vi "Fetch Waveform (Digital Waveform).vi"(4 "Ending Point (10000000)":i32=10000000, 6 "Starting Point (0)":i32, 8 "error in (no error)":errorcluster, 9 "Maximum Time (10000 ms)":u32=10000, 10 "Digital Channel (14: Digital Channel D0)":u16(ring)=14 items=["Digital Channel D0"=14, "Digital Channel D1"=15, "Digital Channel D2"=16, "Digital Channel D3"=17, "Digital Channel D4"=18, "Digital Channel D5"=19, "Digital Channel D6"=20, "Digital Channel D7"=21, "Digital Channel D8"=22, "Digital Channel D9"=23, "Digital Channel D10"=24, "Digital Channel D11"=25, "Digital Channel D12"=26, "Digital Channel D13"=27, "Digital Channel D14"=28, "Digital Channel D15"=29], 11 "VISA resource name":refnum<visa-resource-name>) -> (0 "error out":errorcluster, 2 "Digital Waveform":digitalwaveform(graph), 3 "VISA resource name out":refnum<visa-resource-name>)   [LabVIEW 2017, in "Tektronix DPO MSO 2000 4000 Series.lvlib"]
doc: "Fetches the digital waveform from the chosen digital channel. Please note that it might be necessary to increase the <B>Maximum Time</B> to approximately 170 seconds when fetching waveforms with 10 million data points.\n\n<B>Note:</B> This VI does not check the instrument status. Typically, you call this VI only in a sequence of calls to other low-level instrument driver VIs. The sequence performs one operation. You use the low-level VIs to optimize one or more aspects of interaction with the instrument. If you want to check the instrument status, call the <B>Error Query VI</B> at the conclusion of the sequence.\n\nLabVIEW versions higher than 7.1 might display the data differently."
uses:
  Tektronix DPO MSO 2000 4000 Series.lvlib
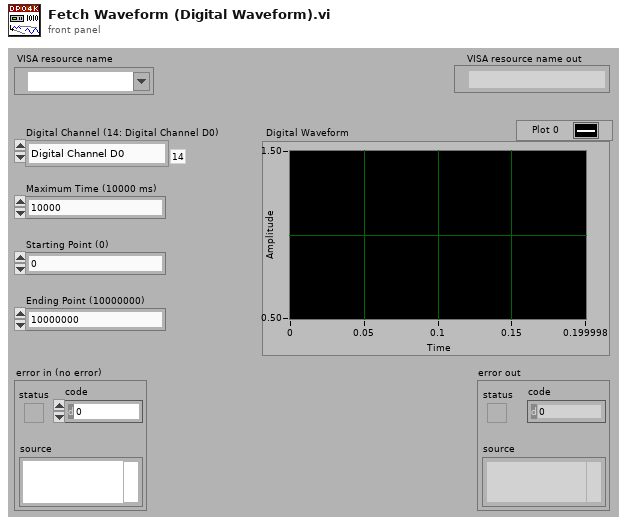
[diagram p1: front panel]
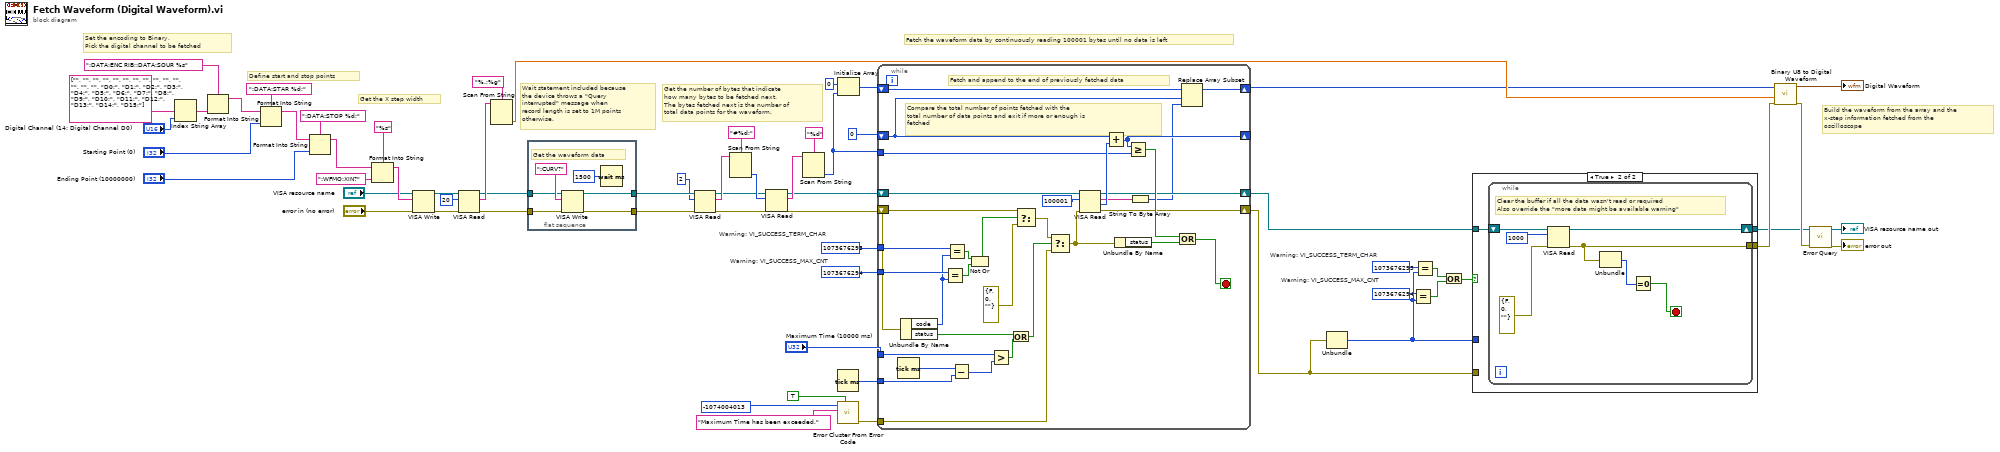
[diagram p0: block diagram]
diagram:
  # "Wait statement included because\nthe device throws a \"Query\ninterrupted\" message when\nrecord length is set to 1M points\notherwise."
  # "Get the number of bytes that indicate\nhow many bytes to be fetched next.\nThe bytes fetched next is the number of\ntotal data points for the waveform."
  # "Define start and stop points"
  # "Warning: VI_SUCCESS_MAX_CNT"
  # "Warning: VI_SUCCESS_TERM_CHAR"
  # "Warning: VI_SUCCESS_MAX_CNT"
  # "Warning: VI_SUCCESS_TERM_CHAR"
  # "Set the encoding to Binary,\nPick the digital channel to be fetched"
  # "Build the waveform from the array and the\nx-step information fetched from the \noscilloscope"
  # "Get the X step width"
  # "Fetch the waveform data by continuously reading 100001 bytes until no data is left"
  n1 = Index String Array(1:"Digital Channel (14: Digital Channel D0)", 2:string[] ["", "", "", "", "", "", "", "", "", "", "", "", "", "", "D0;", "D1;", "D2;", "D3;", "D4;", "D5;", "D6;", "D7;", "D8;", "D9;", "D10;", "D11;", "D12;", "D13;", "D14;", "D15;"]) -> (0:w61:string)  [unwired: 1 in]
  n2 = Format Into String(format string=":DATA:ENC RIB;:DATA:SOUR %s", w61) -> (resulting string=w10:string)  [unwired: 2 in, 1 out]
  n3 = Format Into String(format string=":DATA:STAR %d;", initial string=w10, "Starting Point (0)") -> (resulting string=w9:string)  [unwired: 1 in, 1 out]
  n4 = Format Into String(format string=":DATA:STOP %d;", initial string=w9, "Ending Point (10000000)") -> (resulting string=w8:string)  [unwired: 1 in, 1 out]
  n5 = Format Into String(format string="%s", initial string=w8, ":WFMO:XIN?" ("input 1")) -> (resulting string=w58:string)  [unwired: 1 in, 1 out]
  n6 = VISA Write(VISA resource name="VISA resource name", write buffer=w58, error in (no error)="error in (no error)") -> (VISA resource name out=w54:refnum<visa-resource-name>, error out=w53:errorcluster)  [unwired: 1 out]
  n7 = VISA Read(VISA resource name=w54, byte count=u32 20, error in (no error)=w53) -> (VISA resource name out=w25:refnum<visa-resource-name>, read buffer=w42:string, error out=w26:errorcluster)  [unwired: 1 out]
  n8 = Scan From String(format string="%.;%g", input string=w42) -> (output 1=w3:dbl)  [unwired: 3 in, 3 out]
  n9 = flat-sequence {
    tunnel: [w68] -> w32
    tunnel: [w67] -> w31
    tunnel: w26 -> [w66]
    tunnel: w25 -> [w65]
    frame #0 {
      # "Get the waveform data"
      n10 = VISA Write(VISA resource name=w65, write buffer=":CURV?", error in (no error)=w66) -> (VISA resource name out=w68:refnum<visa-resource-name>, error out=w67:errorcluster)  [unwired: 1 out]
      n11 = Wait (ms)(milliseconds to wait=u32 1500) -> ()  [unwired: 1 out]
    }
  }
  n12 = VISA Read(VISA resource name=w32, byte count=u32 2, error in (no error)=w31) -> (VISA resource name out=w22:refnum<visa-resource-name>, read buffer=w29:string, error out=w21:errorcluster)  [unwired: 1 out]
  n13 = Scan From String(format string="#%d;", input string=w29) -> (output 1=w27:i32)  [unwired: 3 in, 3 out]
  n14 = VISA Read(VISA resource name=w22, byte count=w27, error in (no error)=w21) -> (VISA resource name out=w20:refnum<visa-resource-name>, read buffer=w24:string, error out=w19:errorcluster)  [unwired: 1 out]
  n15 = Scan From String(format string="%d", input string=w24) -> (output 1=w16:i32)  [unwired: 3 in, 3 out]
  n16 = Tick Count (ms)() -> (millisecond timer value=w49:u32)
  n17 = call <vilib>:"Error Cluster From Error Code.vi"("show call chain? (False)"=TRUE, "error message (\"\")"="Maximum Time has been exceeded." ("error message (\"\")"), "error code (0)"=-1074004013) -> ("error out"=w47:errorcluster)  [unwired: 6 in]
  n18 = Initialize Array(0, w16) -> (w18:i32[])
  n19 = while {
    shift-right: [w78] -> w35
    shift-left: w20 -> [w84]
    shift-right: [w79] -> w36
    shift-left: w19 -> [w99]
    tunnel: w16 -> [w71]
    tunnel: 1073676293 -> [w101]
    tunnel: 1073676294 -> [w100]
    tunnel: w49 -> [w93]
    tunnel: "Maximum Time (10000 ms)" -> [w91]
    tunnel: w47 -> [w87]
    shift-right: [w77] -> _
    shift-left: 0 -> [w72]
    shift-right: [w73] -> w1
    shift-left: w18 -> [w74]
    stop <- w85 stop-if-true
    # "Compare the total number of points fetched with the \ntotal number of data points and exit if more or enough is\nfetched"
    # "Fetch and append to the end of previously fetched data"
    n20 = Tick Count (ms)() -> (millisecond timer value=w94:u32)
    n21 = Unbundle By Name(w99) -> ("code"=w98:i32, "status"=w90:bool)
    n22 = Equal?(x=w100, y=w98) -> (x = y?=w96:bool)
    n23 = Equal?(x=w101, y=w98) -> (x = y?=w97:bool)
    n24 = Subtract(x=w94, y=w93) -> (x-y=w92:u32)
    n25 = Not Or(1:w96, 2:w97) -> (0:w95:bool)
    n26 = Greater?(x=w91, y=w92) -> (0:w89:bool)
    n27 = Or(x=w90, y=w89) -> (x .or. y?=w88:bool)
    n28 = Select(t=w99, s=w95, f=errorcluster {"status"=FALSE, "code"=0, "source"=""}) -> (s? t:f=w83:errorcluster)
    n29 = Select(t=w83, s=w88, f=w87) -> (s? t:f=w70:errorcluster)
    n30 = VISA Read(VISA resource name=w84, byte count=u32 100001, error in (no error)=w70) -> (VISA resource name out=w78:refnum<visa-resource-name>, read buffer=w76:string, return count=w81:u32, error out=w79:errorcluster)
    n31 = Add(x=w72, y=w81) -> (x+y=w77:u32)
    n32 = Unbundle By Name(w70) -> ("status"=w86:bool)
    n33 = Greater Or Equal?(x=w77, y=w71) -> (x >= y?=w80:bool)
    n34 = String To Byte Array(string=w76) -> (unsigned byte array=w75:u8[])
    n35 = Compound Arithmetic op=OR(w80, w86) -> (w85:bool)
    n36 = Replace Array Subset(array=w74, new element=w75, index=w72) -> (w73:i32[])
  }
  n37 = Unbundle(w36) -> ("code"=w33:i32)  [unwired: 2 out]
  n38 = Equal?(x=1073676294, y=w33) -> (x = y?=w34:bool)
  n39 = Equal?(x=1073676293, y=w33) -> (x = y?=w40:bool)
  n40 = Or(x=w40, y=w34) -> (x .or. y?=w39:bool)
  n41 = case shown="True" w39 {
    tunnel: w36 -> [w103 _]
    tunnel: w35 -> [w104 w106]
    tunnel: [w104 w105] -> w4
    tunnel: [w103 w107] -> w15
    tunnel: w33 -> [_ _]
    frame False {
      # "Buffer Clear or there is another error present,\npass it forward."
    }
    frame True {
      n42 = while {
        shift-right: [w112] -> w105
        shift-left: w106 -> [w113]
        tunnel: [w111] -> w107
        stop <- w108 stop-if-true
        # "Clear the buffer if all the data wasn't read or required\nAlso override the \"more data might be available warning\""
        n43 = VISA Read(VISA resource name=w113, byte count=u32 1000, error in (no error)=errorcluster {"status"=FALSE, "code"=0, "source"=""}) -> (VISA resource name out=w112:refnum<visa-resource-name>, error out=w111:errorcluster)  [unwired: 2 out]
        n44 = Unbundle(w111) -> ("code"=w109:i32)  [unwired: 2 out]
        n45 = Equal To 0?(x=w109) -> (x = 0?=w108:bool)
      }
    }
  }
  n46 = call "Binary U8 to Digital Waveform.vi"("error in (no error)"=w15, "Time Division (0.0001 s)"=w3, "Binary Array"=w1) -> ("error out"=w5:errorcluster, "Digital Waveform Graph"=→"Digital Waveform":digitalwaveform)  [unwired: 7 in]
  n47 = call "Error Query.vi"("error in (no error)"=w5, "VISA resource name"=w4) -> ("error out"=→"error out":errorcluster, "VISA resource name out"=→"VISA resource name out":refnum<visa-resource-name>)  [unwired: 6 in, 2 out]
